vi "Request Task Run Info.vi"(8 "error in (no error)":errorcluster, 11 "VolatusAPI in":refnum<class "VolatusAPI.lvclass">) -> (0 "error out":errorcluster, 2 "Task Run Info":T1[](array[typedef]), 3 "VolatusAPI out":refnum<class "VolatusAPI.lvclass">)   [LabVIEW 2020, in "Volatus.lvlib" / "VolatusAPI.lvclass"]
uses:
  VolatusAPI.lvclass
  VolatusAPI.lvclass/VolatusAPI.ctl
  lv-promises/Promises/Promise/Promise.lvclass
  TaskRunInfoArrayValue/TaskRunInfoArrayValue.lvclass
  VolatusCore Messages/Request Task Run Info Msg/Request Task Run Info Msg.lvclass
  lv-promises/Promises/Future/Future.lvclass
  C:/dev/lv20CE/relink/lv-promises/Promises/Value/Value.lvclass
  C:/dev/lv20CE/relink/lv-volatus/Volatus/TaskRunInfoArrayValue/TaskRunInfoArrayValue.lvclass
  Task Hierarchy.ctl
  Volatus.lvlib
  Task State.ctl
  Task Run Info.ctl
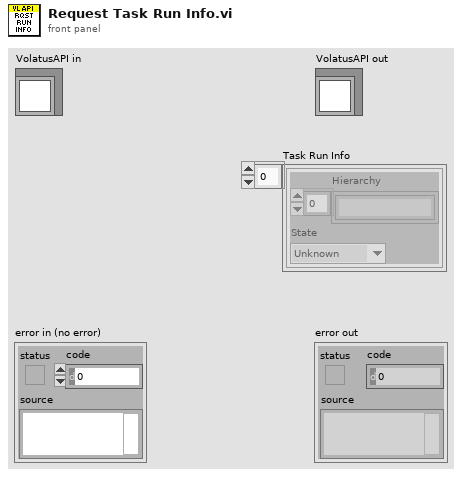
[diagram p1: front panel]
types:
  T1 = typedef "Volatus.lvlib/Task Run Info.ctl" = cluster{"Hierarchy":T2, "State":T3}
  T2 = typedef "Volatus.lvlib/Task Hierarchy.ctl" = string[]
  T3 = typedef "Volatus.lvlib/Task State.ctl" = enum16{"Unknown", "Idle", "Initializing", "Starting", "Running", "Stopping", "Stopped", "Error - Init", "Error - Start", "Error - Run", "Error - Stop"}
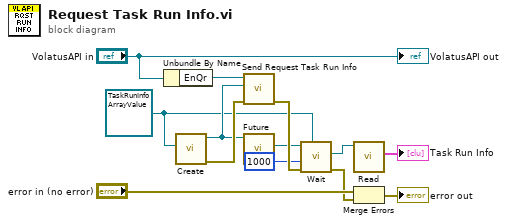
[diagram p0: block diagram]
diagram:
  w5 = refnum<class "TaskRunInfoArrayValue.lvclass"> refnum ("Volatus:TaskRunInfoArrayValue.lvclass")
  n1 = Unbundle By Name("VolatusAPI in") -> ("EnQr"=w10:refnum<class "Message Enqueuer.lvclass">)
  n2 = call "Create.vi"("Result Type"=w5) -> ("error out"=w9:errorcluster, "Promise"=w8:refnum<class "Promise.lvclass">)  [unwired: 9 in]
  n3 = call "Send Request Task Run Info.vi"("error in (no error)"=w9, "Promise"=w8, "Message Enqueuer"=w10) -> ("error out"=w13:errorcluster)  [unwired: 7 in, 1 out]
  n4 = call "Future.vi"("Promise in"=w8) -> ("Future"=w7:refnum<class "Future.lvclass">)  [unwired: 9 in, 1 out]
  n5 = call "Wait.vi"("Result Type"=w5, "error in (no error)"=w13, "Timeout mS (-1)"=1000, "Future in"=w7) -> ("error out"=w1:errorcluster, "Result"=w4:refnum<class "TaskRunInfoArrayValue.lvclass">)  [unwired: 6 in]
  n6 = call "Read.vi"("TaskRunInfoArrayValue in"=w4) -> ("Task Run Info"=→"Task Run Info":T1[])  [unwired: 10 in]
  n7 = Merge Errors("error in (no error)", w1) -> (→"error out":errorcluster)
  "VolatusAPI out" <- "VolatusAPI in"
